vi "MH_BuffAndQDeltasB.vi"(6 "queue out":refnum<queue>, 7 "DeltasBuffer":i32[](array[numeric]), 8 "erroIn":errorcluster caption="error In") -> (0 "error out":errorcluster)   [LabVIEW 2019]
uses:
  <userlib>/MultiHarp150/T2Lib/MH_T2DeltaQMessage.ctl
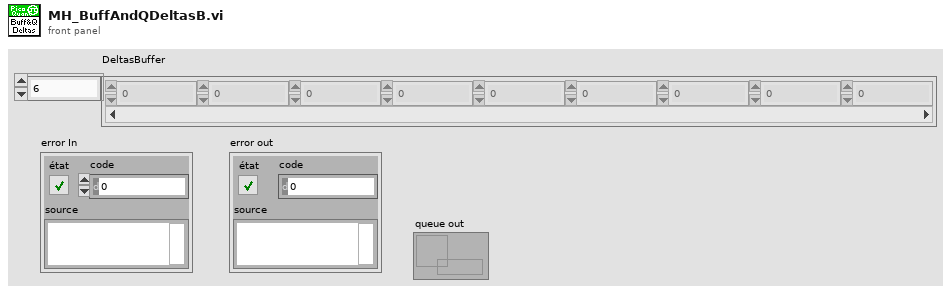
[diagram p1: front panel]
types:
  T1 = typedef "MH_T2DeltaQMessage.ctl" = cluster{"Message":string, "buffer":i32[], "Code":i32, "nactual":i32}
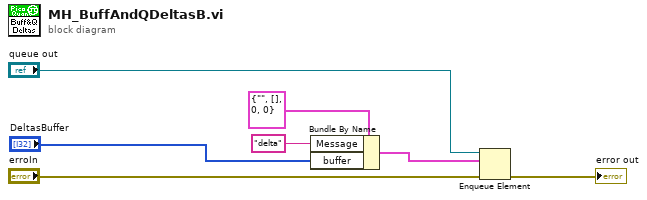
[diagram p0: block diagram]
diagram:
  n1 = Bundle By Name(cluster=T1 {"Message"="", "buffer"=[], "Code"=0, "nactual"=0} ("ClassQueue"), "Message"="delta", "buffer"="DeltasBuffer") -> (w2:T1)
  n2 = Enqueue Element(queue="queue out", element=w2, error in (no error)="erroIn") -> (error out=→"error out":errorcluster)  [unwired: 1 in, 2 out]
